vi "VelocityControl.vi"() -> ()   [LabVIEW 2024]
uses:
  <vilib>/Analysis/Matrix/Datatypes/RealMatrix.ctl
  GitHub/ME121-25/LabVIEW/SerialVIs/subs/portX.xctl
  <vilib>/Analysis/baseanly.llb/A x Vector.vi
  <vilib>/Analysis/baseanly.llb/Real Inverse Matrix.vi
  <vilib>/Analysis/NI_AALBase.lvlib
  <vilib>/Analysis/Matrix/NI_Matrix.lvlib
panel:
  out "Array 2":dbl[](array[numeric])
  out "Array":dbl[](array[numeric])
  out "resulting string":string
  in  "portX":refnum<visa-resource-name>(xcontrol)
  in  "qs":dbl[](array[numeric])
  out "2D Picture":picture
  out "Inverse J":T1
  in  "L2":dbl=75.0
  in  "L1":dbl=75.0
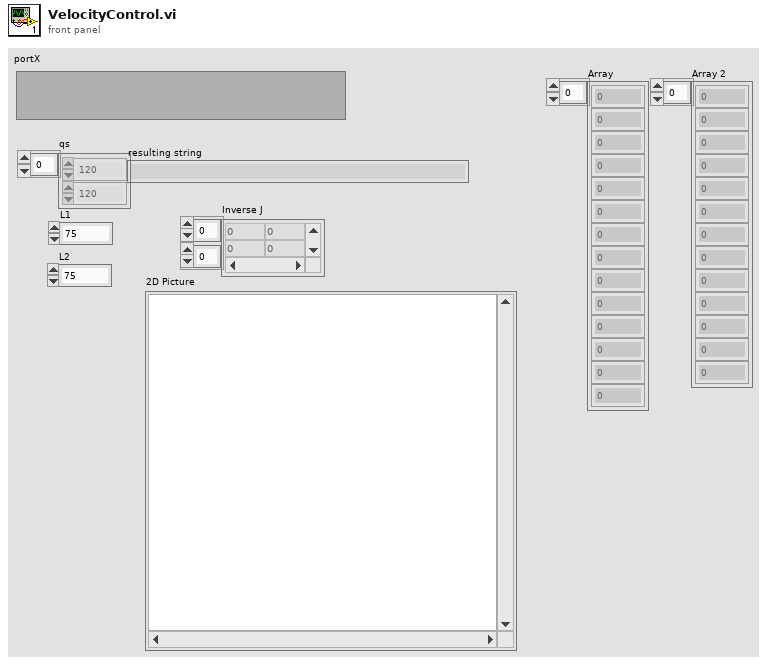
[diagram p1: front panel]
types:
  T1 = typedef "NI_Matrix.lvlib/RealMatrix.ctl" = dbl[][]
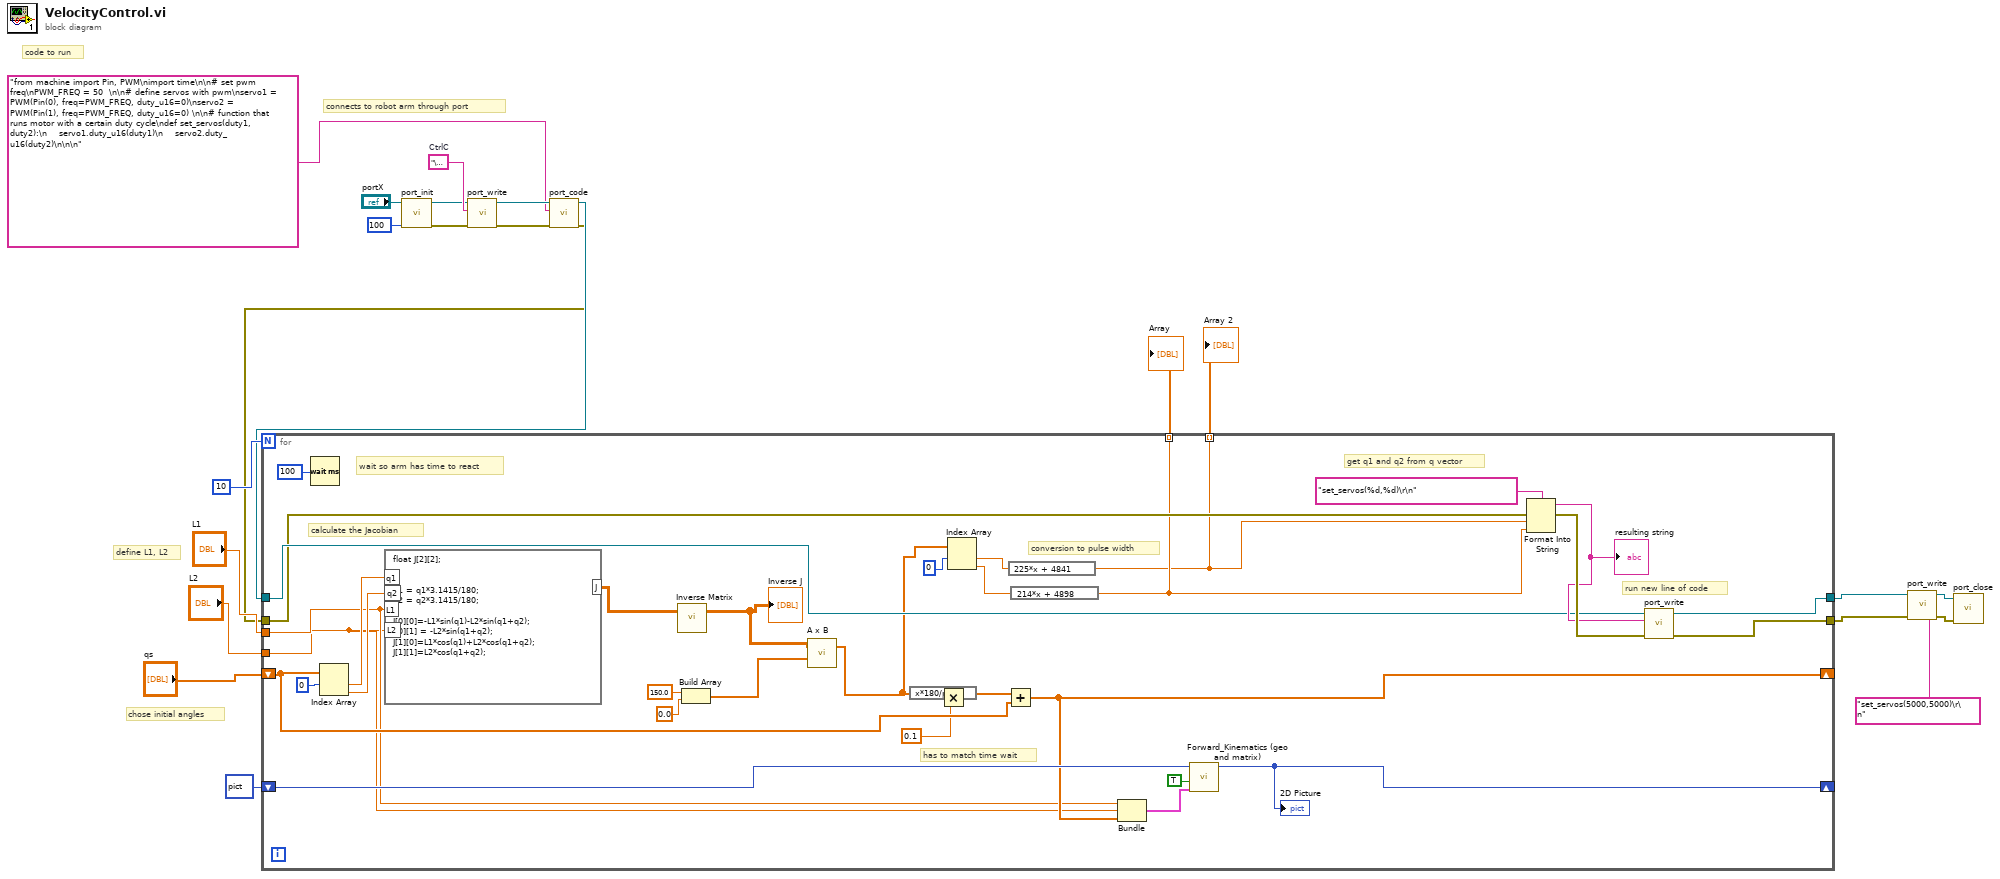
[diagram p0: block diagram]
diagram:
  w18 = "\u0003"  # CtrlC
  # "code to run"
  # "connects to robot arm through port"
  # "chose initial angles"
  # "define L1, L2"
  n1 = call "port_init.vi"("Timeout (ms)"=u32 100, "VISA Refnum in"="portX") -> ("error out"=w16:errorcluster, "VISA Refnum out"=w17:refnum<visa-resource-name>)  [unwired: 8 in]
  n2 = call "port_write.vi"("error in (no error)"=w16, "write buffer"=w18, "VISA Refnum in"=w17) -> ("error out"=w12:errorcluster, "VISA Refnum out"=w13:refnum<visa-resource-name>)  [unwired: 7 in]
  n3 = call "port_code.vi"("error in (no error)"=w12, "Code to run"="from machine import Pin, PWM\nimport time\n\n# set pwm freq\nPWM_FREQ = 50  \n\n# define servos with pwm\nservo1 = PWM(Pin(0), freq=PWM_FREQ, duty_u16=0)\nservo2 = PWM(Pin(1), freq=PWM_FREQ, duty_u16=0) \n\n# function that runs motor with a certain duty cycle\ndef set_servos(duty1, duty2):\n    servo1.duty_u16(duty1)\n    servo2.duty_u16(duty2)\n\n\n", "VISA Refnum in"=w13) -> ("error out"=w8:errorcluster, "VISA Refnum out"=w9:refnum<visa-resource-name>)  [unwired: 7 in]
  n4 = for {
    N: 10 -> [_]
    tunnel: "L1" -> [w38]
    tunnel: "L2" -> [w37]
    shift-right: [w43] -> _
    shift-left: "qs" -> [w44]
    shift-right: [w39] -> _
    shift-left: picture data[5B] ("2D Picture") -> [w49]
    tunnel: w9 -> [w29]
    tunnel: [w30] -> w7
    tunnel: w8 -> [w28]
    tunnel: [w31] -> w5
    tunnel: [w26] -> w2 mode=indexing
    tunnel: [w25] -> w1 mode=indexing
    # "has to match time wait"
    # "get q1 and q2 from q vector"
    # "run new line of code"
    # "wait so arm has time to react"
    # "conversion to pulse width"
    # "calculate the Jacobian"
    n5 = Wait (ms)(milliseconds to wait=u32 100) -> ()  [unwired: 1 out]
    n6 = Index Array "Index Array"(array=w44, index #1=0 ("index (row)")) -> (element #1=w52:dbl, element #2=w48:dbl)  [unwired: 1 in]
    n7 = formula code="float J[2][2];\n\n\nq1 = q1*3.1415/180;\nq2 = q2*3.1415/180;\n\nJ[0][0]=-L1*sin(q1)-L2*sin(q1+q2);\nJ[0][1] = -L2*sin(q1+q2);\nJ[1][0]=L1*cos(q1)+L2*cos(q1+q2);\nJ[1][1]=L2*cos(q1+q2);"("q1"=w52, "q2"=w48, "L1"=w38, "L2"=w37) -> ("J"=w55:dbl[][])
    n8 = call-poly <vilib>:"Inverse Matrix.vi"("Input Matrix"=w55) -> ("Inverse Matrix"=w51:T1)  [unwired: 1 in, 1 out]
    "Inverse J" <- w51
    n9 = Build Array(150.0 ("element"), 0.0 ("element")) -> (w46:dbl[])
    n10 = call-poly <vilib>:"A x B.vi"("Vector"=w46, "A"=w51) -> ("A x Vector"=w27:dbl[])  [unwired: 1 out]
    n11 = expression code="x*180/pi"(w27) -> (w24:dbl[])
    n12 = Multiply ("Multiply.vi")(x=w24, y=0.1) -> (x*y=w45:dbl[])
    n13 = Index Array "Index Array"(array=w27, index #1=0 ("index (row)")) -> (element #1=w35:dbl, element #2=w23:dbl)  [unwired: 1 in]
    n14 = Add(x=w45, y=w44) -> (x+y=w43:dbl[])
    n15 = expression code="225*x + 4841"(w35) -> (w25:dbl)
    n16 = expression code="214*x + 4898"(w23) -> (w26:dbl)
    n17 = Bundle("L1"=w38, "L2"=w37, w43) -> (w50:cluster{"L1":dbl, "L2":dbl, dbl[]})  [unwired: 1 in]
    n18 = call "Forward_Kinematics (geo and matrix).vi"("geometry"=w50, "geometry?"=TRUE, "picture in"=w49) -> ("2D Picture"=w39:picture)  [unwired: 6 in, 2 out]
    "2D Picture" <- w39
    n19 = Format Into String "Format Into String"(format string="set_servos(%d,%d)\r\n", error in=w28, w25, w26) -> (resulting string=w32:string, error out=w33:errorcluster)  [unwired: 1 in]
    "resulting string" <- w32
    n20 = call "port_write.vi"("error in (no error)"=w33, "write buffer"=w32, "VISA Refnum in"=w29) -> ("error out"=w31:errorcluster, "VISA Refnum out"=w30:refnum<visa-resource-name>)  [unwired: 7 in]
  }
  "Array" <- w2
  "Array 2" <- w1
  n21 = call "port_write.vi"("error in (no error)"=w5, "write buffer"="set_servos(5000,5000)\r\n", "VISA Refnum in"=w7) -> ("error out"=w4:errorcluster, "VISA Refnum out"=w6:refnum<visa-resource-name>)  [unwired: 7 in]
  n22 = call "port_close.vi"("error in (no error)"=w4, "VISA Refnum in"=w6) -> ()  [unwired: 10 in]
